vi "Write ParameterOptions.vi"(8 "error in (no error)":errorcluster, 10 "ParameterOptions":T1(array[cluster]) {"Direction" items=["Input"=1, "Output"=2, "InputOutput"=3, "ReturnValue"=6]; "DbType" items=["AnsiString"=0, "Binary"=1, "Byte"=2, "Boolean"=3, "Currency"=4, "Date"=5, "DateTime"=6, "Decimal"=7, "Double"=8, "Guid"=9, "Int16"=10, "Int32"=11, "Int64"=12, "Object"=13, "SByte"=14, "Single"=15, "String"=16, "Time"=17, "UInt16"=18, "UInt32"=19, "UInt64"=20, "VarNumeric"=21, "AnsiStringFixedLength"=22, "StringFixedLength"=23, "Xml"=25, "DateTime2"=26, "DateTimeOffset"=27]}, 11 "DynamicParameters in":refnum<class "DynamicParameters.lvclass">) -> (0 "error out":errorcluster, 3 "DynamicParameters out":refnum<class "DynamicParameters.lvclass">)   [LabVIEW 2020, in "ORM.lvlib" / "DynamicParameters.lvclass"]
uses:
  DynamicParameters.lvclass
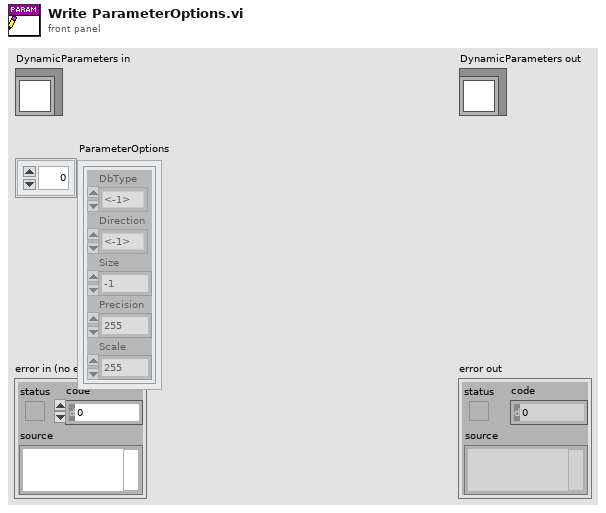
[diagram p1: front panel]
types:
  T1 = cluster{"DbType":i32, "Direction":i32, "Size":i32, "Precision":u8, "Scale":u8}[]
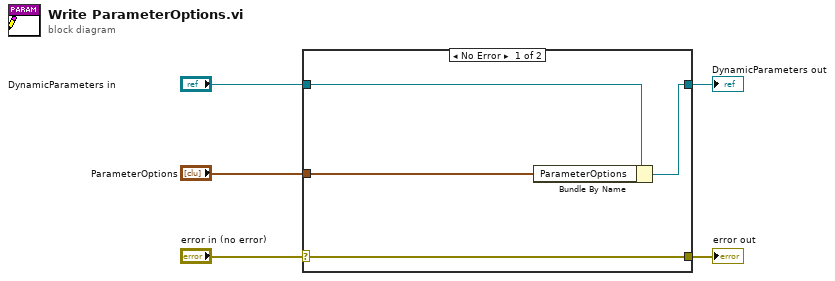
[diagram p0: block diagram]
diagram:
  n1 = case shown="No Error" "error in (no error)" {
    selector: "error in (no error)" -> [w9 w10]
    tunnel: [w9 w10] -> w4
    tunnel: [w7 w11] -> w2
    tunnel: "DynamicParameters in" -> [w8 w11]
    tunnel: "ParameterOptions" -> [w6 _]
    frame No Error {
      n2 = Bundle By Name(cluster=w8, "ParameterOptions"=w6) -> (w7:refnum<class "DynamicParameters.lvclass">)
    }
    frame Error {
    }
  }
  "error out" <- w4
  "DynamicParameters out" <- w2
